vi "UCTGetOffset.vi"() -> (0 "Local UCT Offset String":string, 1 "Local UCT Offset (sec)":i32)   [LabVIEW 2010]
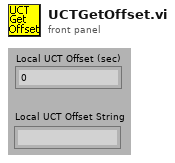
[diagram p1: front panel]
types:
  T1 = cluster{"second":i32, "minute":i32, "hour":i32, "day of month":i32, "month":i32, "year":i32, "day of week":i32, "day of year":i32, "is DST":i32}
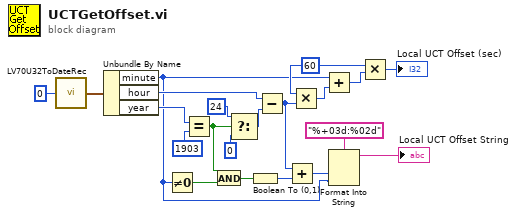
[diagram p0: block diagram]
diagram:
  w17 = 60
  n1 = call <vilib>:"LV70U32ToDateRec.vi"("Time"=u32 0 ("secondes écoulées")) -> ("date time rec"=w20:T1)
  n2 = Unbundle By Name(w20) -> ("minute"=w3:i32, "hour"=w15:i32, "year"=w12:i32)
  n3 = Not Equal To 0?(x=w3) -> (x != 0?=w9:bool)
  n4 = Equal?(x=w12, y=1903) -> (x = y?=w8:bool)
  n5 = And(x=w8, y=w9) -> (x .and. y?=w7:bool)
  n6 = Select(t=24, s=w8, f=0) -> (s? t:f=w14:i32)
  n7 = Boolean To (0,1)(Boolean=w7) -> (0, 1=w6:i16)
  n8 = Subtract(x=w15, y=w14) -> (x-y=w5:i32)
  n9 = Add(x=w5, y=w6) -> (x+y=w4:i32)
  n10 = Multiply(x=w17, y=w5) -> (x*y=w19:i32)
  n11 = Add(x=w3, y=w19) -> (x+y=w18:i32)
  n12 = Format Into String(format string="%+03d:%02d" ("chaîne de format"), w4, w3) -> (resulting string=→"Local UCT Offset String":string)  [unwired: 2 in, 1 out]
  n13 = Multiply(x=w17, y=w18) -> (x*y=→"Local UCT Offset (sec)":i32)
